vi "Time_elapsed.vi"(4 "End of previous average in":dbl, 6 "New Scan Index?":bool, 7 "Averaging time (mins)":dbl format="%.2f") -> (0 "End of previous average out":dbl, 1 "End of period":dbl, 2 "Start of period":dbl, 3 "Take new reading?":bool)   [LabVIEW 2015]
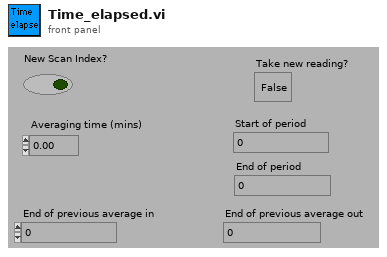
[diagram p1: front panel]
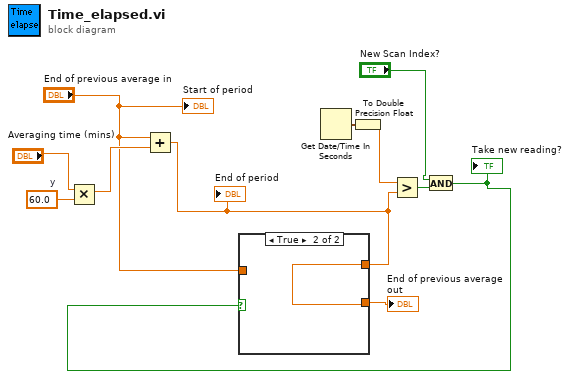
[diagram p0: block diagram]
diagram:
  w11 = 60.0  # y
  n1 = Multiply(x="Averaging time (mins)", y=w11) -> (x*y=w9:dbl)
  n2 = Add(x="End of previous average in", y=w9) -> (x+y=w5:dbl)
  "End of period" <- w5
  n3 = Get Date/Time In Seconds() -> (seconds since 1Jan1904=w4:timestamp)
  n4 = To Double Precision Float(number=w4) -> (double precision float=w8:dbl)
  n5 = Greater?(x=w8, y=w5) -> (0:w3:bool)
  n6 = And(x="New Scan Index?", y=w3) -> (x .and. y?=w1:bool)
  "Take new reading?" <- w1
  n7 = case shown="True" w1 {
    tunnel: [w12 w13] -> w7
    tunnel: "End of previous average in" -> [w12 _]
    tunnel: w5 -> [_ w13]
    frame False {
    }
    frame True {
    }
  }
  "End of previous average out" <- w7
  "Start of period" <- "End of previous average in"
